vi "Random Number (Range) U32.vi"(1 "lower bound":u32, 2 "upper bound":u32=100) -> (0 "number":u32)   [LabVIEW 2016, in "Simple Tester.lvclass"]
doc: "This VI generate a random U32 value within the specified range.\n\nThis VI is a copy of the \"sub_Random U32.vi\" vi.lib VI that is present in the latest versions of LabVIEW.\n\nThis copy was created because the sub_Random U32.vi does not exist in the LabVIEW 2016 vi.lib."
uses:
  Simple Tester.lvclass
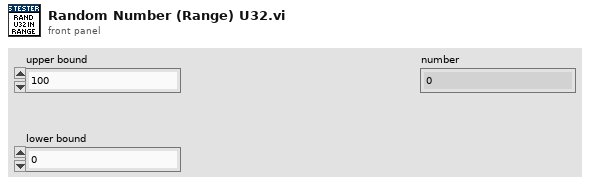
[diagram p1: front panel]
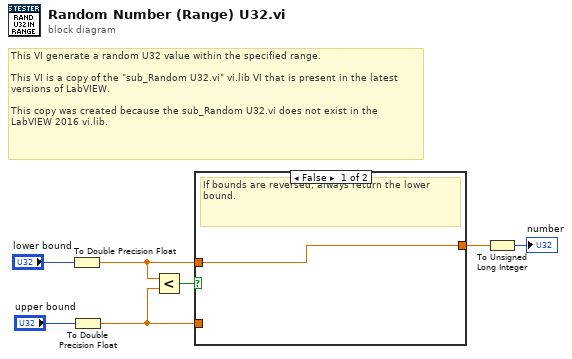
[diagram p0: block diagram]
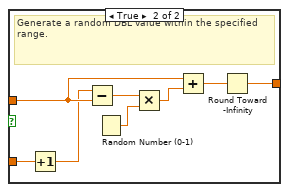
[diagram p2: hidden frame]
diagram:
  # "This VI generate a random U32 value within the specified range.\n\nThis VI is a copy of the \"sub_Random U32.vi\" vi.lib VI that is present in the latest versions of LabVIEW.\n\nThis copy was created because the sub_Random U32.vi does not exist in the LabVIEW 2016 vi.lib."
  n1 = To Double Precision Float(number="lower bound") -> (double precision float=w3:dbl)
  n2 = To Double Precision Float(number="upper bound") -> (double precision float=w2:dbl)
  n3 = Less?(x=w3, y=w2) -> (x < y?=w7:bool)
  n4 = case shown="False" w7 {
    tunnel: w3 -> [w8 w13]
    tunnel: w2 -> [_ w16]
    tunnel: [w8 w9] -> w4
    frame False {
      # "If bounds are reversed, always return the lower bound."
    }
    frame True {
      # "Generate a random DBL value within the specified range."
      n5 = Increment(x=w16) -> (x+1=w10:dbl)
      n6 = Subtract(x=w10, y=w13) -> (x-y=w15:dbl)
      n7 = Random Number (0-1)() -> (number: 0 to 1=w14:dbl)
      n8 = Multiply(x=w15, y=w14) -> (x*y=w12:dbl)
      n9 = Add(x=w13, y=w12) -> (x+y=w11:dbl)
      n10 = Round Toward -Infinity(1:w11) -> (0:w9:dbl)
    }
  }
  n11 = To Unsigned Long Integer(number=w4) -> (unsigned 32bit integer=→"number":u32)
